vi "New Set Camera Mode Message.vi"() -> (0 "Set Camera Mode Message":T1)   [LabVIEW 2016]
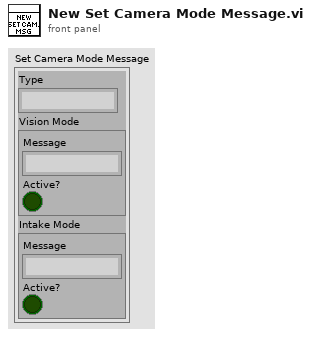
[diagram p1: front panel]
types:
  T1 = cluster{"Type":string, "Vision Mode":cluster{"Message":string, "Active?":bool}, "Intake Mode":cluster{"Message":string, "Active?":bool}}
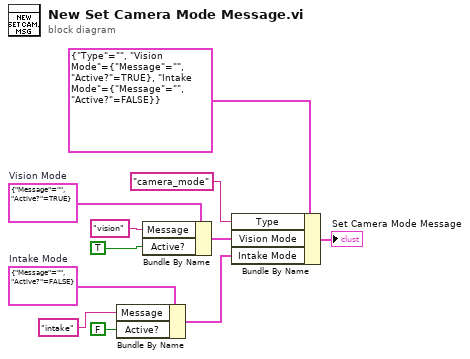
[diagram p0: block diagram]
diagram:
  w5 = cluster{"Message":string, "Active?":bool} {"Message"="", "Active?"=FALSE}  # Intake Mode
  w9 = cluster{"Message":string, "Active?":bool} {"Message"="", "Active?"=TRUE}  # Vision Mode
  n1 = Bundle By Name(cluster=w5, "Message"="intake", "Active?"=FALSE) -> (w2:cluster{"Message":string, "Active?":bool})
  n2 = Bundle By Name(cluster=w9, "Message"="vision", "Active?"=TRUE) -> (w6:cluster{"Message":string, "Active?":bool})
  n3 = Bundle By Name(cluster=T1 {"Type"="", "Vision Mode"={"Message"="", "Active?"=TRUE}, "Intake Mode"={"Message"="", "Active?"=FALSE}}, "Type"="camera_mode", "Vision Mode"=w6, "Intake Mode"=w2) -> (→"Set Camera Mode Message":T1)
